vi "Execute.vi"(5 "SleepTerminalArray":refnum<vi>, 6 "ExeRef":refnum<vi>, 7 "ActiveTerminalArray":refnum<vi>, 8 "error in (no error)":errorcluster, 9 "Json_In":string, 10 "VariableRef":T2, 11 "Info":T1) -> (0 "Error Out":errorcluster, 1 "NumResultArray":dbl[](array[numeric]), 2 "StrResultArray":string[](array[string]), 3 "StrResult":string, 4 "NumResult":dbl)   [LabVIEW 2018, in "String.lvlib"]
uses:
  String.lvlib
  <userlib>/_OpenG.lib/dictionary/dictionary.llb/Dictionary Object RefNum__ogtk.ctl
  <userlib>/_OpenG.lib/dictionary/dictionary.llb/Dictionary Object RefNum - Enum__ogtk.ctl
  <vilib>/Utility/error.llb/whitespace.ctl
  <userlib>/_OpenG.lib/md5/md5.llb/MD5 Message Digest (Hexadecimal String)__ogtk.vi
  <vilib>/regexp/Match Regular Expression.xnode
  <vilib>/addons/_JKI.lib/Serialization/JSON/JKI JSON Serialization.lvlib
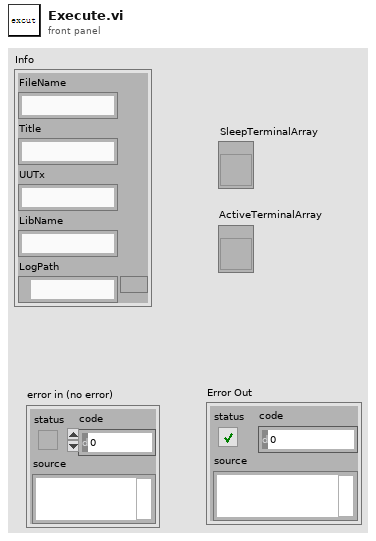
[diagram p1: front panel]
types:
  T1 = cluster{"FileName":string, "Title":string, "UUTx":string, "LibName":string, "LogPath":path}
  T2 = typedef "Dictionary Object RefNum__ogtk.ctl" = refnum<k1>
  T3 = cluster{"StringLength":cluster{"json":cluster{"Method":string, "StringVar":string}}, "InitialString":cluster{"json":cluster{"Method":string, "Strings":string}}, "StringSubset":cluster{"json":cluster{"Method":string, "StringVar":string, "offset":i32, "length":i32}}, "TrimWhitespace":cluster{"json":cluster{"Method":string, "StringVar":string, "Location":string}}, "ReplaceSubstring":cluster{"json":cluster{"Method":string, "StringVar":string, "Substring":string, "Offset":i32, "Length":i32}}, "SearchandReplaceString":cluster{"json":cluster{"Method":string, "StringVar":string, "SearchString":string, "Offset":i32, "ReplaceString":string, "ReplaceAll":bool, "IgnoreCase":bool}}, "MatchPattern":cluster{"json":cluster{"Method":string, "StringVar":string, "RegularExpression ":string, "Offset":i32}}, "MatchRegularExpression":cluster{"json":cluster{"Method":string, "StringVar":string, "RegularExpression ":string, "Offset":i32, "IgnoreCase":bool, "Multiline":bool}}, "FormatDate/TimeString":cluster{"json":cluster{"Method":string, "TimeFormatString ":string, "UTCFormat":bool}}, "ToLowerCase":cluster{"json":cluster{"Method":string, "StringVar":string}}, "ToUpperCase":cluster{"json":cluster{"Method":string, "StringVar":string}}, "StringMD5":cluster{"json":cluster{"Method":string, "StringVar":string}}, "NumStringToHexString":cluster{"json":cluster{"Method":string, "StringVar":string}}, "HexStringToNumString":cluster{"json":cluster{"Method":string, "StringVar":string}}, "StartWith":cluster{"json":cluster{"Method":string, "StringVar":string, "SubString":string, "IgnoreCasse":bool}}, "EndWith":cluster{"json":cluster{"Method":string, "StringVar":string, "SubString":string, "IgnoreCasse":bool}}, "AfterSubstring":cluster{"json":cluster{"Method":string, "StringVar":string, "SubString":string}}, "BeforeSubstring":cluster{"json":cluster{"Method":string, "StringVar":string, "SubString":string}}, "MiddleSubstring":cluster{"json":cluster{"Method":string, "StringVar":string, "BeforeSubString":string, "AfterSubString":string}}, "AsciiToHexString":cluster{"json":cluster{"Method":string, "StringVar":string}}, "HexStringToAscii":cluster{"json":cluster{"Method":string, "StringVar":string}}, "StringTo1DArray":cluster{"json":cluster{"Method":string, "StringVar":string, "Delimiter":string}}, "StringToCharacterArray":cluster{"json":cluster{"Method":string, "StringVar":string}}, "RemoveAllWhitespace":cluster{"json":cluster{"Method":string, "StringVar":string}}}
  T4 = cluster{"json":cluster{"Method":string, "StringVar":string}}
  T5 = cluster{"json":cluster{"Method":string, "Strings":string}}
  T6 = cluster{"json":cluster{"Method":string, "StringVar":string, "offset":i32, "length":i32}}
  T7 = cluster{"json":cluster{"Method":string, "StringVar":string, "Location":string}}
  T8 = typedef "whitespace.ctl" = u16
  T9 = cluster{"json":cluster{"Method":string, "StringVar":string, "Substring":string, "Offset":i32, "Length":i32}}
  T10 = cluster{"json":cluster{"Method":string, "StringVar":string, "SearchString":string, "Offset":i32, "ReplaceString":string, "ReplaceAll":bool, "IgnoreCase":bool}}
  T11 = cluster{"json":cluster{"Method":string, "StringVar":string, "RegularExpression ":string, "Offset":i32}}
  T12 = cluster{"json":cluster{"Method":string, "StringVar":string, "RegularExpression ":string, "Offset":i32, "IgnoreCase":bool, "Multiline":bool}}
  T13 = cluster{"json":cluster{"Method":string, "TimeFormatString ":string, "UTCFormat":bool}}
  T14 = cluster{"json":cluster{"Method":string, "StringVar":string, "SubString":string, "IgnoreCasse":bool}}
  T15 = cluster{"json":cluster{"Method":string, "StringVar":string, "SubString":string}}
  T16 = cluster{"json":cluster{"Method":string, "StringVar":string, "BeforeSubString":string, "AfterSubString":string}}
  T17 = cluster{"json":cluster{"Method":string, "StringVar":string, "Delimiter":string}}
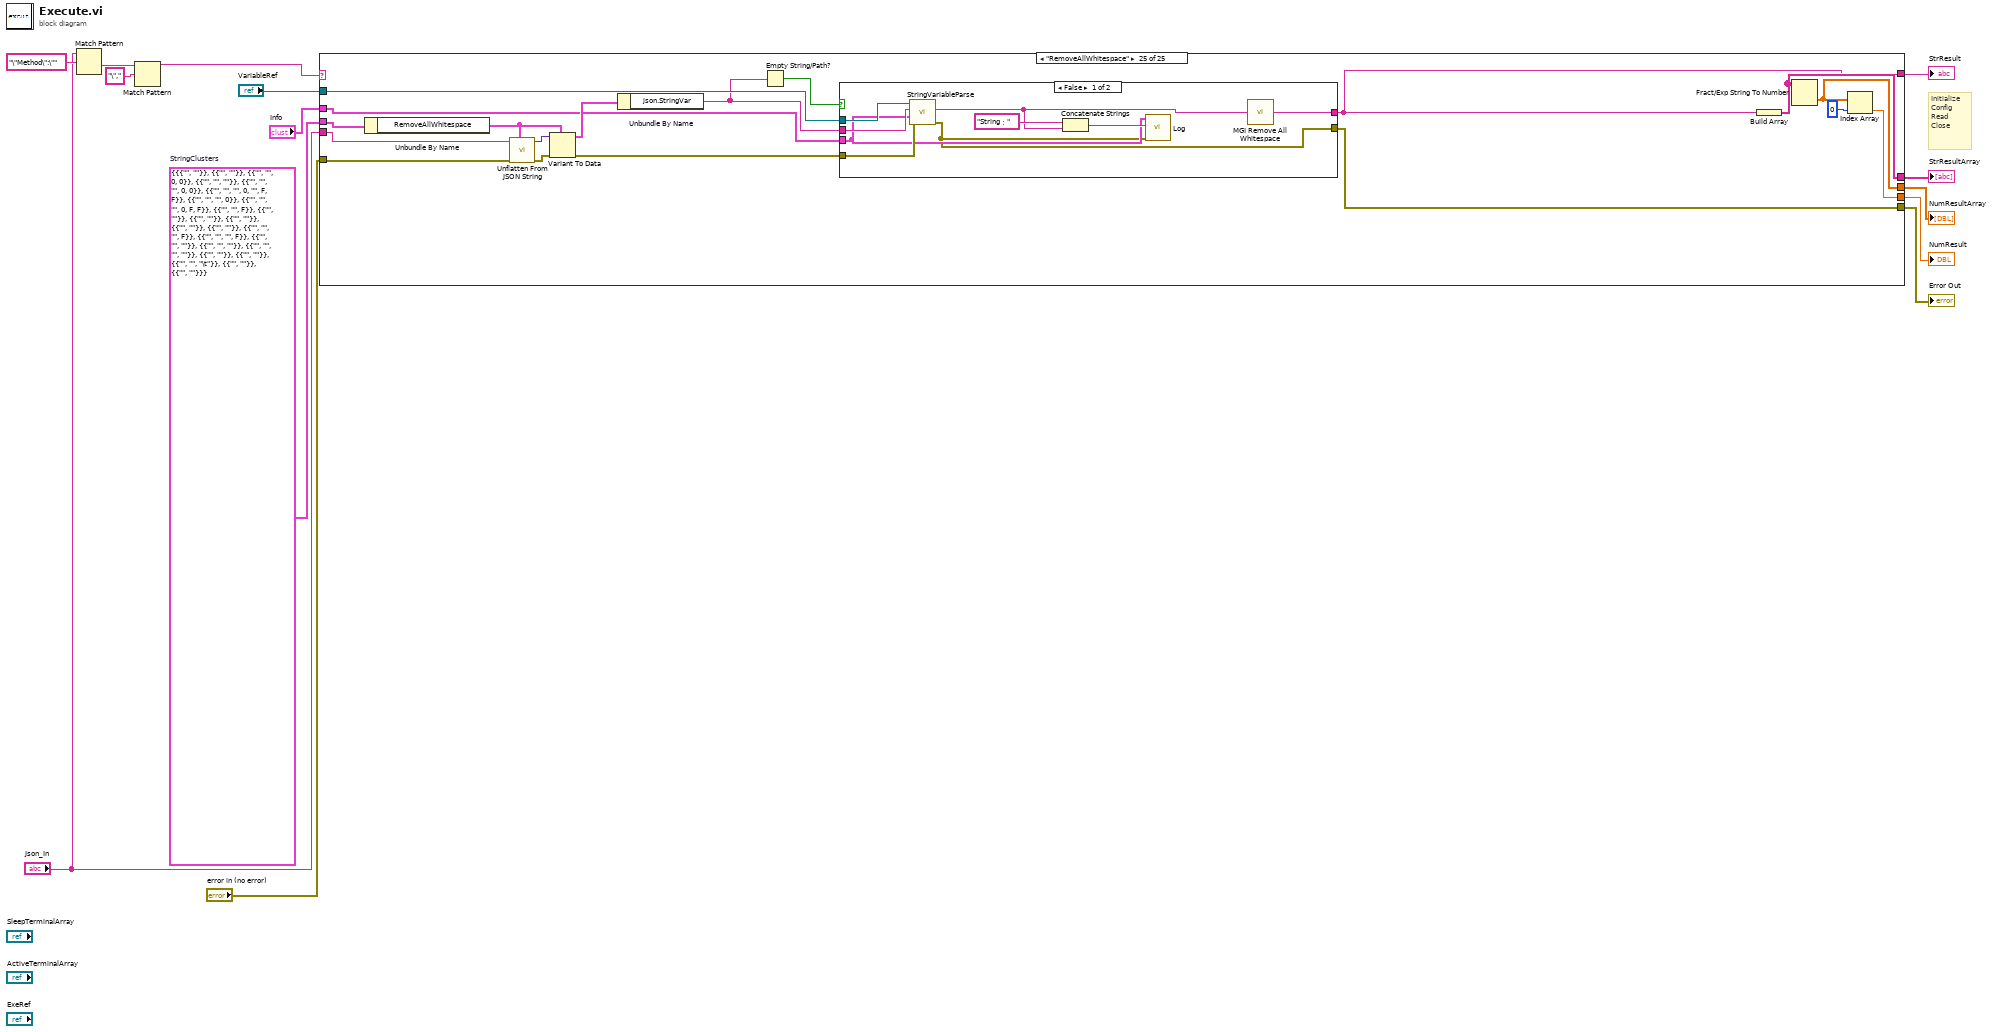
[diagram p0: block diagram]
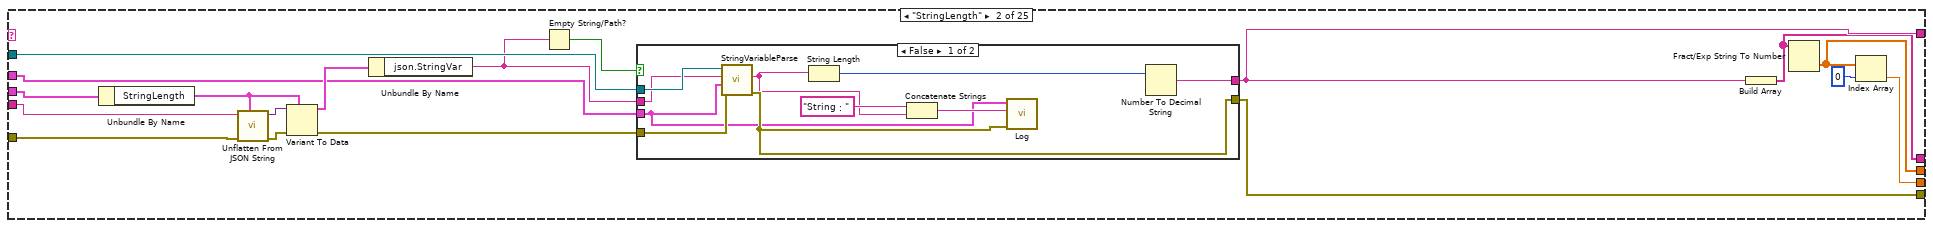
[diagram p3: hidden frame]
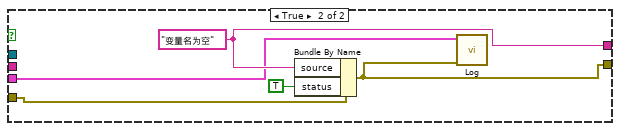
[diagram p4: hidden frame]
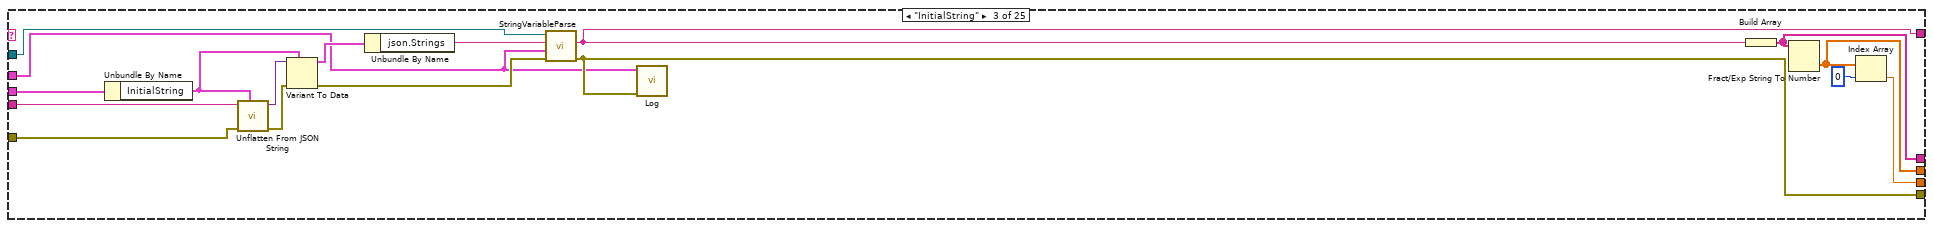
[diagram p5: hidden frame]
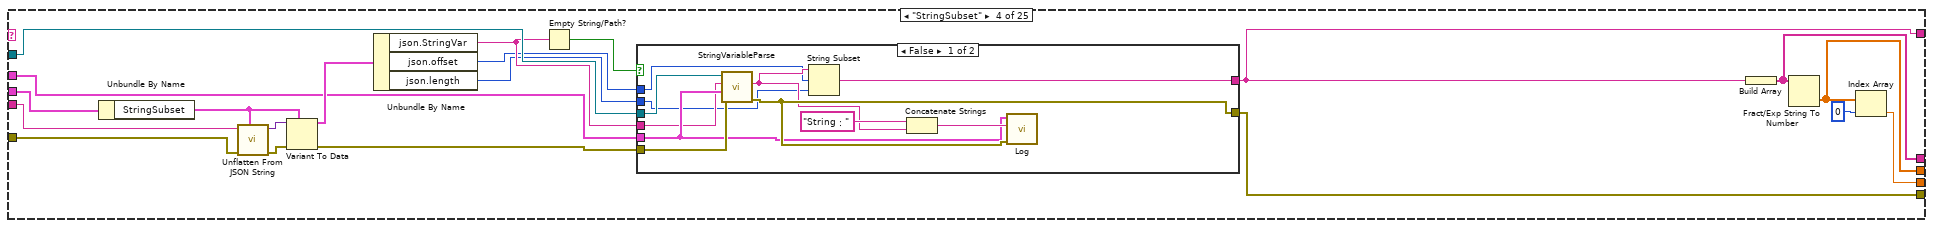
[diagram p6: hidden frame]
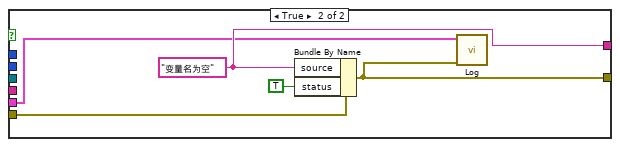
[diagram p7: hidden frame]
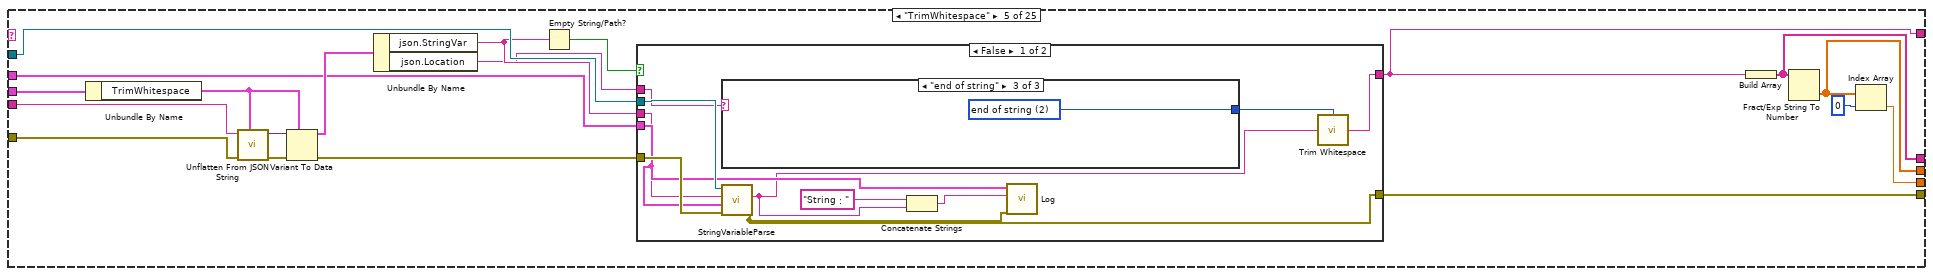
[diagram p8: hidden frame]
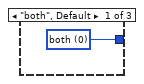
[diagram p9: hidden frame]
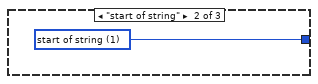
[diagram p10: hidden frame]
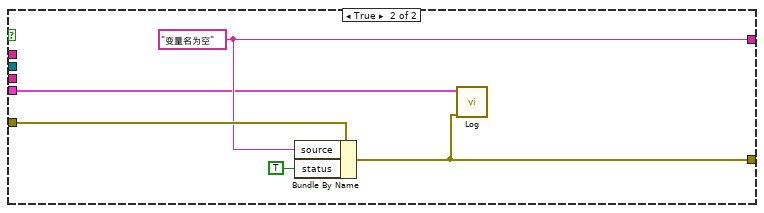
[diagram p11: hidden frame]
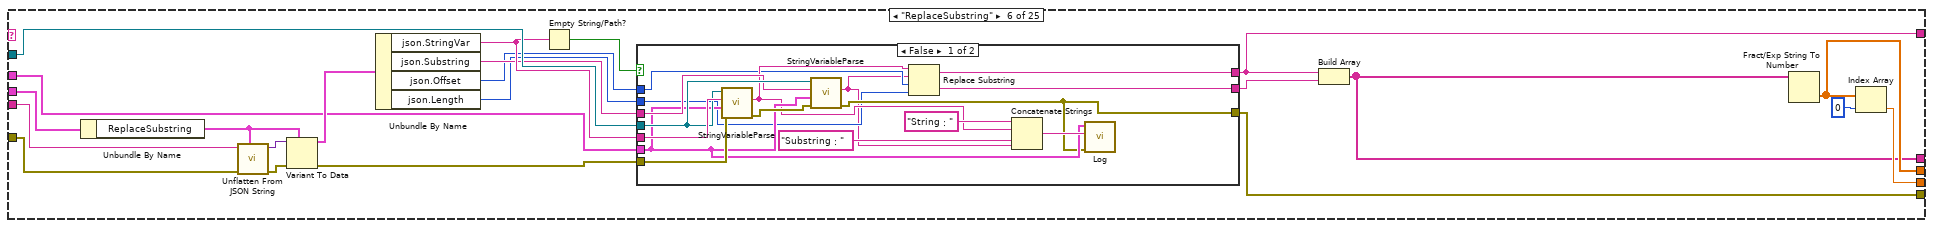
[diagram p12: hidden frame]
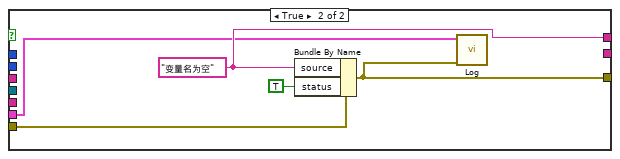
[diagram p13: hidden frame]
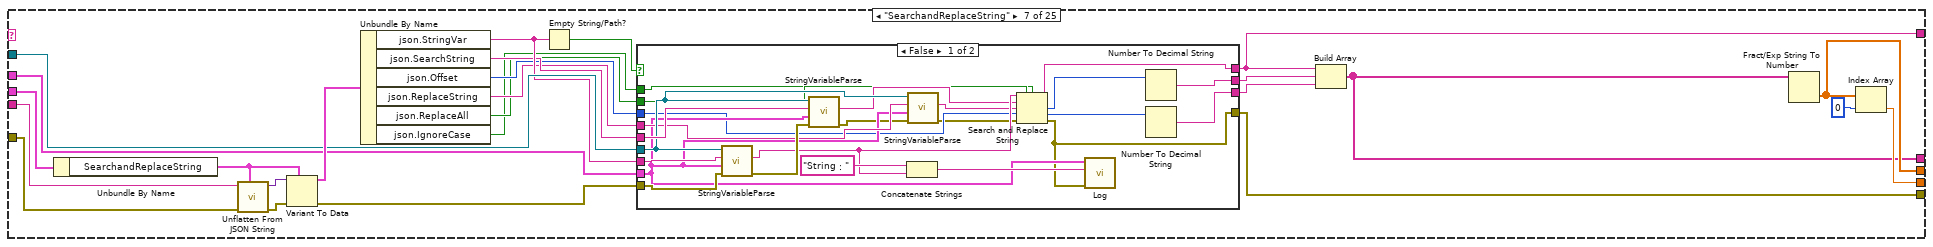
[diagram p14: hidden frame]
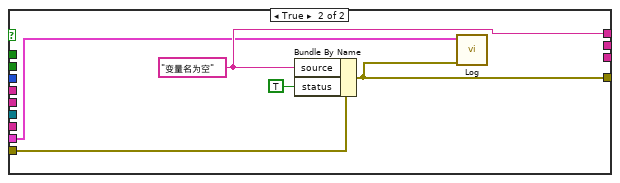
[diagram p15: hidden frame]
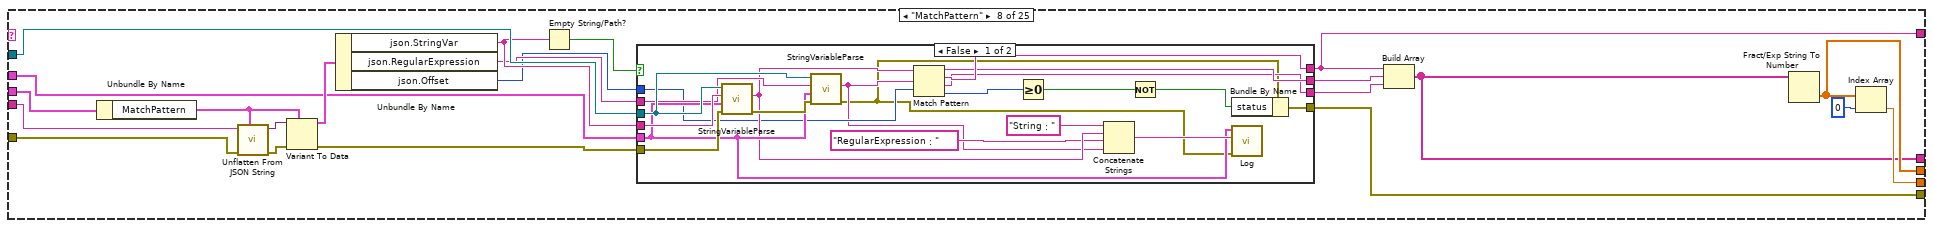
[diagram p16: hidden frame]
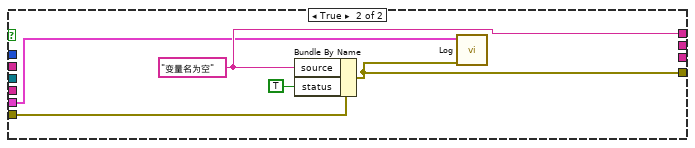
[diagram p17: hidden frame]
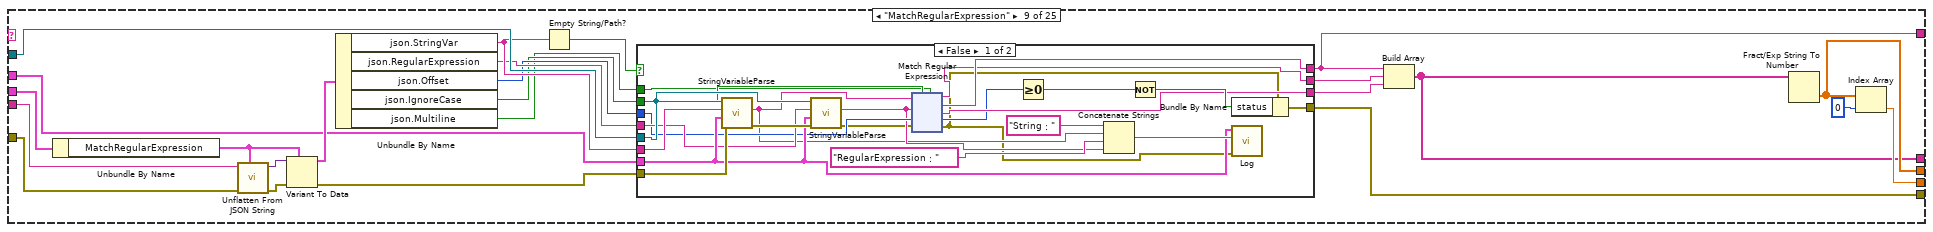
[diagram p18: hidden frame]
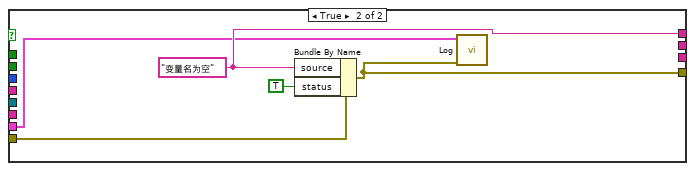
[diagram p19: hidden frame]
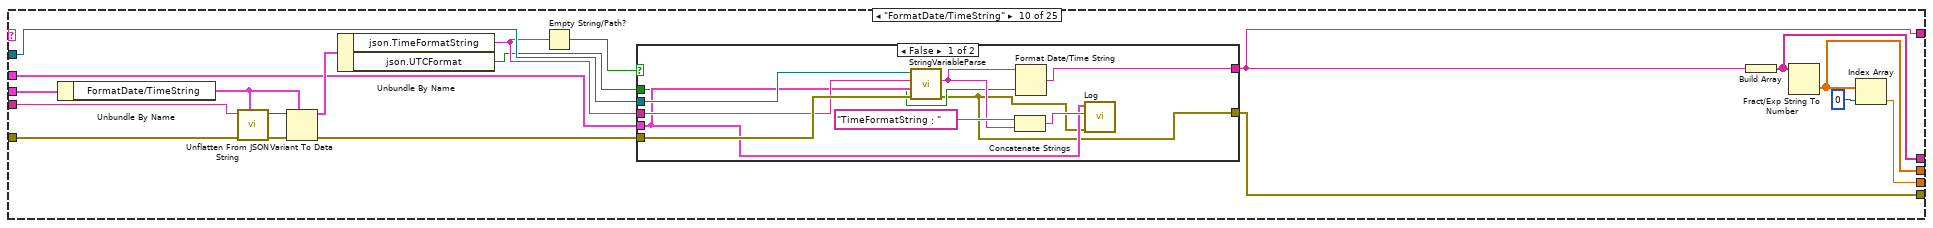
[diagram p20: hidden frame]
diagram:
  w1 = T3 {"StringLength"={"json"={"Method"="", "StringVar"=""}}, "InitialString"={"json"={"Method"="", "Strings"=""}}, "StringSubset"={"json"={"Method"="", "StringVar"="", "offset"=0, "length"=0}}, "TrimWhitespace"={"json"={"Method"="", "StringVar"="", "Location"=""}}, "ReplaceSubstring"={"json"={"Method"="", "StringVar"="", "Substring"="", "Offset"=0, "Length"=0}}, "SearchandReplaceString"={"json"={"Method"="", "StringVar"="", "SearchString"="", "Offset"=0, "ReplaceString"="", "ReplaceAll"=FALSE, "IgnoreCase"=FALSE}}, "MatchPattern"={"json"={"Method"="", "StringVar"="", "RegularExpression "="", "Offset"=0}}, "MatchRegularExpression"={"json"={"Method"="", "StringVar"="", "RegularExpression "="", "Offset"=0, "IgnoreCase"=FALSE, "Multiline"=FALSE}}, "FormatDate/TimeString"={"json"={"Method"="", "TimeFormatString "="", "UTCFormat"=FALSE}}, "ToLowerCase"={"json"={"Method"="", "StringVar"=""}}, "ToUpperCase"={"json"={"Method"="", "StringVar"=""}}, "StringMD5"={"json"={"Method"="", "StringVar"=""}}, "NumStringToHexString"={"json"={"Method"="", "StringVar"=""}}, "HexStringToNumString"={"json"={"Method"="", "StringVar"=""}}, "StartWith"={"json"={"Method"="", "StringVar"="", "SubString"="", "IgnoreCasse"=FALSE}}, "EndWith"={"json"={"Method"="", "StringVar"="", "SubString"="", "IgnoreCasse"=FALSE}}, "AfterSubstring"={"json"={"Method"="", "StringVar"="", "SubString"=""}}, "BeforeSubstring"={"json"={"Method"="", "StringVar"="", "SubString"=""}}, "MiddleSubstring"={"json"={"Method"="", "StringVar"="", "BeforeSubString"="", "AfterSubString"=""}}, "AsciiToHexString"={"json"={"Method"="", "StringVar"=""}}, "HexStringToAscii"={"json"={"Method"="", "StringVar"=""}}, "StringTo1DArray"={"json"={"Method"="", "StringVar"="", "Delimiter"="\t"}}, "StringToCharacterArray"={"json"={"Method"="", "StringVar"=""}}, "RemoveAllWhitespace"={"json"={"Method"="", "StringVar"=""}}}  # StringClusters
  # "Initialize\nConfig\nRead\nClose"
  n1 = Match Pattern(string="Json_In", regular expression="\"Method\":\"") -> (after substring=w4:string)  [unwired: 1 in, 3 out]
  n2 = Match Pattern(string=w4, regular expression="\",") -> (before substring=w2:string)  [unwired: 1 in, 3 out]
  n3 = case shown="\"RemoveAllWhitespace\"" w2 {
    tunnel: "Json_In" -> [_ w30 w62 w82 w117 w158 w204 w254 w303 w464 w497 w529 w561 w593 w626 w661 w821 w980 w1016 w1053 w1103 w1150 w1194 w1231 w1264]
    tunnel: [w15 w25 w58 w66 w102 w144 w190 w240 w289 w450 w483 w515 w547 w579 w612 w647 w807 w966 w1004 w1041 w1091 w1138 w1182 w1219 w1252] -> w14
    tunnel: "error in (no error)" -> [w15 w29 w61 w81 w116 w157 w203 w253 w302 w463 w496 w528 w560 w592 w625 w660 w820 w979 w1015 w1052 w1102 w1149 w1193 w1230 w1263]
    tunnel: [_ w17 w49 w67 w103 w145 w191 w241 w290 w451 w484 w516 w548 w580 w613 w648 w808 w967 w1002 w1037 w1089 w1136 w1180 w1218 w1250] -> w12
    tunnel: "VariableRef" -> [_ w27 w59 w73 w108 w149 w195 w245 w294 w455 w488 w520 w552 w584 w617 w652 w812 w971 w1008 w1045 w1095 w1142 w1186 w1223 w1256]
    tunnel: [_ w16 w50 w75 w110 w151 w197 w247 w296 w457 w490 w522 w554 w586 w619 w654 w814 w973 w1001 w1038 w1090 w1137 w1179 w1217 w1251] -> w11
    tunnel: [_ w20 w53 w78 w113 w154 w200 w250 w299 w460 w493 w525 w557 w589 w622 w657 w817 w976 w1012 w1049 w1099 w1146 w1190 w1227 w1260] -> w10
    tunnel: [_ w22 w55 w80 w115 w156 w202 w252 w301 w462 w495 w527 w559 w591 w624 w659 w819 w978 w1014 w1051 w1101 w1148 w1192 w1229 w1262] -> w9
    tunnel: "Info" -> [_ w23 w56 w70 w105 w146 w192 w242 w291 w452 w485 w517 w549 w581 w614 w649 w809 w968 w1005 w1042 w1092 w1139 w1183 w1220 w1253]
    tunnel: w1 -> [_ w19 w52 w77 w112 w153 w199 w249 w298 w459 w492 w524 w556 w588 w621 w656 w816 w975 w1011 w1048 w1098 w1145 w1189 w1226 w1259]
    frame Default {
    }
    frame "StringLength" {
      n4 = Unbundle By Name(w19) -> ("StringLength"=w18:T4)
      n5 = call <vilib>:"Unflatten From JSON String.vi"("Type and Defaults"=w18, "error in (no error)"=w29, "JSON String"=w30) -> ("error out"=w32:errorcluster, "Variant"=w33:variant)  [unwired: 7 in]
      n6 = Variant To Data(error in=w32, type=w18, Variant=w33) -> (data=w31:T4, error out=w28:errorcluster)
      n7 = Unbundle By Name(w31) -> ("json.StringVar"=w24:string)
      n8 = Empty String/Path?(string/path=w24) -> (empty?=w26:bool)
      n9 = case shown="False" w26 {
        tunnel: w28 -> [w43 w48]
        tunnel: w27 -> [w42 _]
        tunnel: [w41 w44] -> w25
        tunnel: w24 -> [w38 _]
        tunnel: [w34 w46] -> w17
        tunnel: w23 -> [w39 w45]
        frame False {
          n10 = call "StringVariableParse.vi"("error in"=w43, "Info"=w39, "in"=w38, "dictionary"=w42) -> ("error out"=w41:errorcluster, "out"=w36:string)  [unwired: 5 in, 1 out]
          n11 = String Length(string=w36) -> (length=w35:i32)
          n12 = Concatenate Strings("String：" ("string"), w36) -> (w40:string)
          n13 = call "Log.vi"("error in"=w41, "LogIn"=w40, "Info"=w39) -> ()  [unwired: 9 in]
          n14 = Number To Decimal String(number=w35) -> (decimal integer string=w34:string)  [unwired: 1 in]
        }
        frame True {
          w46 = "变量名为空" ("source")
          n15 = Bundle By Name(cluster=w48, "source"=w46, "status"=TRUE) -> (w44:errorcluster)
          n16 = call "Log.vi"("error in"=w44, "Info"=w45) -> ()  [unwired: 10 in]
        }
      }
      n17 = Build Array(w17) -> (w16:string[])
      n18 = Fract/Exp String To Number(string=w16) -> (number=w22:dbl[])  [unwired: 3 in, 1 out]
      n19 = Index Array(array=w22, index=0) -> (element=w20:dbl)
    }
    frame "InitialString" {
      n20 = Unbundle By Name(w52) -> ("InitialString"=w51:T5)
      n21 = call <vilib>:"Unflatten From JSON String.vi"("Type and Defaults"=w51, "error in (no error)"=w61, "JSON String"=w62) -> ("error out"=w64:errorcluster, "Variant"=w65:variant)  [unwired: 7 in]
      n22 = Variant To Data(error in=w64, type=w51, Variant=w65) -> (data=w63:T5, error out=w60:errorcluster)
      n23 = Unbundle By Name(w63) -> ("json.Strings"=w57:string)
      n24 = call "StringVariableParse.vi"("error in"=w60, "Info"=w56, "in"=w57, "dictionary"=w59) -> ("error out"=w58:errorcluster, "out"=w49:string)  [unwired: 5 in, 1 out]
      n25 = call "Log.vi"("error in"=w58, "Info"=w56) -> ()  [unwired: 10 in]
      n26 = Build Array(w49) -> (w50:string[])
      n27 = Fract/Exp String To Number(string=w50) -> (number=w55:dbl[])  [unwired: 3 in, 1 out]
      n28 = Index Array(array=w55, index=0) -> (element=w53:dbl)
    }
    frame "StringSubset" {
      n29 = Unbundle By Name(w77) -> ("StringSubset"=w76:T6)
      n30 = call <vilib>:"Unflatten From JSON String.vi"("Type and Defaults"=w76, "error in (no error)"=w81, "JSON String"=w82) -> ("error out"=w84:errorcluster, "Variant"=w85:variant)  [unwired: 7 in]
      n31 = Variant To Data(error in=w84, type=w76, Variant=w85) -> (data=w83:T6, error out=w71:errorcluster)
      n32 = Unbundle By Name(w83) -> ("json.StringVar"=w72:string, "json.offset"=w69:i32, "json.length"=w68:i32)
      n33 = Empty String/Path?(string/path=w72) -> (empty?=w74:bool)
      n34 = case shown="False" w74 {
        tunnel: w71 -> [w96 w101]
        tunnel: w73 -> [w95 _]
        tunnel: [w94 w97] -> w66
        tunnel: w72 -> [w91 _]
        tunnel: [w86 w99] -> w67
        tunnel: w70 -> [w92 w98]
        tunnel: w69 -> [w88 _]
        tunnel: w68 -> [w87 _]
        frame False {
          n35 = call "StringVariableParse.vi"("error in"=w96, "Info"=w92, "in"=w91, "dictionary"=w95) -> ("error out"=w94:errorcluster, "out"=w89:string)  [unwired: 5 in, 1 out]
          n36 = String Subset(string=w89, offset (0)=w88, length (rest)=w87) -> (substring=w86:string)
          n37 = Concatenate Strings("String：" ("string"), w89) -> (w93:string)
          n38 = call "Log.vi"("error in"=w94, "LogIn"=w93, "Info"=w92) -> ()  [unwired: 9 in]
        }
        frame True {
          w99 = "变量名为空" ("source")
          n39 = Bundle By Name(cluster=w101, "source"=w99, "status"=TRUE) -> (w97:errorcluster)
          n40 = call "Log.vi"("error in"=w97, "Info"=w98) -> ()  [unwired: 10 in]
        }
      }
      n41 = Build Array(w67) -> (w75:string[])
      n42 = Fract/Exp String To Number(string=w75) -> (number=w80:dbl[])  [unwired: 3 in, 1 out]
      n43 = Index Array(array=w80, index=0) -> (element=w78:dbl)
    }
    frame "TrimWhitespace" {
      n44 = Unbundle By Name(w112) -> ("TrimWhitespace"=w111:T7)
      n45 = call <vilib>:"Unflatten From JSON String.vi"("Type and Defaults"=w111, "error in (no error)"=w116, "JSON String"=w117) -> ("error out"=w119:errorcluster, "Variant"=w120:variant)  [unwired: 7 in]
      n46 = Variant To Data(error in=w119, type=w111, Variant=w120) -> (data=w118:T7, error out=w106:errorcluster)
      n47 = Unbundle By Name(w118) -> ("json.StringVar"=w107:string, "json.Location"=w104:string)
      n48 = Empty String/Path?(string/path=w107) -> (empty?=w109:bool)
      n49 = case shown="False" w109 {
        tunnel: w106 -> [w131 w139]
        tunnel: w108 -> [w130 _]
        tunnel: [w129 w135] -> w102
        tunnel: w107 -> [w126 _]
        tunnel: [w124 w137] -> w103
        tunnel: w105 -> [w127 w136]
        tunnel: w104 -> [w121 _]
        frame False {
          n50 = case shown="\"end of string\"" w121 {
            tunnel: [w132 w133 w134] -> w122
            frame "both", Default {
              w132 = T8 0 items=["both", "start of string", "end of string"] ("location (both)")
            }
            frame "start of string" {
              w133 = T8 1 items=["both", "start of string", "end of string"] ("location (both)")
            }
            frame "end of string" {
              w134 = T8 2 items=["both", "start of string", "end of string"] ("location (both)")
            }
          }
          n51 = call "StringVariableParse.vi"("error in"=w131, "Info"=w127, "in"=w126, "dictionary"=w130) -> ("error out"=w129:errorcluster, "out"=w123:string)  [unwired: 5 in, 1 out]
          n52 = Concatenate Strings("String：" ("string"), w123) -> (w128:string)
          n53 = call "Log.vi"("error in"=w129, "LogIn"=w128, "Info"=w127) -> ()  [unwired: 9 in]
          n54 = call <vilib>:"Trim Whitespace.vi"("string"=w123, "location (both)"=w122) -> ("trimmed string"=w124:string)
        }
        frame True {
          w137 = "变量名为空" ("source")
          n55 = Bundle By Name(cluster=w139, "source"=w137, "status"=TRUE) -> (w135:errorcluster)
          n56 = call "Log.vi"("error in"=w135, "Info"=w136) -> ()  [unwired: 10 in]
        }
      }
      n57 = Build Array(w103) -> (w110:string[])
      n58 = Fract/Exp String To Number(string=w110) -> (number=w115:dbl[])  [unwired: 3 in, 1 out]
      n59 = Index Array(array=w115, index=0) -> (element=w113:dbl)
    }
    frame "ReplaceSubstring" {
      n60 = Unbundle By Name(w153) -> ("ReplaceSubstring"=w152:T9)
      n61 = call <vilib>:"Unflatten From JSON String.vi"("Type and Defaults"=w152, "error in (no error)"=w157, "JSON String"=w158) -> ("error out"=w160:errorcluster, "Variant"=w161:variant)  [unwired: 7 in]
      n62 = Variant To Data(error in=w160, type=w152, Variant=w161) -> (data=w159:T9, error out=w147:errorcluster)
      n63 = Unbundle By Name(w159) -> ("json.StringVar"=w148:string, "json.Substring"=w143:string, "json.Offset"=w142:i32, "json.Length"=w141:i32)
      n64 = Empty String/Path?(string/path=w148) -> (empty?=w150:bool)
      n65 = case shown="False" w150 {
        tunnel: w147 -> [w177 w182]
        tunnel: w149 -> [w172 _]
        tunnel: [w169 w178] -> w144
        tunnel: w148 -> [w175 _]
        tunnel: [w165 w180] -> w145
        tunnel: w146 -> [w170 w179]
        tunnel: w143 -> [w171 _]
        tunnel: w142 -> [w167 _]
        tunnel: w141 -> [w166 _]
        tunnel: [w162 _] -> w140
        frame False {
          n66 = call "StringVariableParse.vi"("error in"=w177, "Info"=w170, "in"=w175, "dictionary"=w172) -> ("error out"=w173:errorcluster, "out"=w168:string)  [unwired: 5 in, 1 out]
          n67 = call "StringVariableParse.vi"("error in"=w173, "Info"=w170, "in"=w171, "dictionary"=w172) -> ("error out"=w169:errorcluster, "out"=w163:string)  [unwired: 5 in, 1 out]
          n68 = Replace Substring(2:w166, 3:w167, 4:w163, 5:w168) -> (0:w162:string, 1:w165:string)
          n69 = Concatenate Strings("String：" ("string"), w168, "Substring：" ("string"), w163) -> (w176:string)
          n70 = call "Log.vi"("error in"=w169, "LogIn"=w176, "Info"=w170) -> ()  [unwired: 9 in]
        }
        frame True {
          w180 = "变量名为空" ("source")
          n71 = Bundle By Name(cluster=w182, "source"=w180, "status"=TRUE) -> (w178:errorcluster)
          n72 = call "Log.vi"("error in"=w178, "Info"=w179) -> ()  [unwired: 10 in]
        }
      }
      n73 = Build Array(w145, w140) -> (w151:string[])
      n74 = Fract/Exp String To Number(string=w151) -> (number=w156:dbl[])  [unwired: 3 in, 1 out]
      n75 = Index Array(array=w156, index=0) -> (element=w154:dbl)
    }
    frame "SearchandReplaceString" {
      n76 = Unbundle By Name(w199) -> ("SearchandReplaceString"=w198:T10)
      n77 = call <vilib>:"Unflatten From JSON String.vi"("Type and Defaults"=w198, "error in (no error)"=w203, "JSON String"=w204) -> ("error out"=w206:errorcluster, "Variant"=w207:variant)  [unwired: 7 in]
      n78 = Variant To Data(error in=w206, type=w198, Variant=w207) -> (data=w205:T10, error out=w193:errorcluster)
      n79 = Unbundle By Name(w205) -> ("json.StringVar"=w194:string, "json.SearchString"=w189:string, "json.Offset"=w188:i32, "json.ReplaceString"=w187:string, "json.ReplaceAll"=w186:bool, "json.IgnoreCase"=w185:bool)
      n80 = Empty String/Path?(string/path=w194) -> (empty?=w196:bool)
      n81 = case shown="False" w196 {
        tunnel: w193 -> [w230 w235]
        tunnel: w195 -> [w224 _]
        tunnel: [w212 w231] -> w190
        tunnel: w194 -> [w228 _]
        tunnel: [w214 w233] -> w191
        tunnel: w192 -> [w222 w232]
        tunnel: w189 -> [w225 _]
        tunnel: w188 -> [w217 _]
        tunnel: w187 -> [w223 _]
        tunnel: w186 -> [w216 _]
        tunnel: w185 -> [w215 _]
        tunnel: [w209 _] -> w184
        tunnel: [w208 _] -> w183
        frame False {
          n82 = call "StringVariableParse.vi"("error in"=w230, "Info"=w222, "in"=w228, "dictionary"=w224) -> ("error out"=w226:errorcluster, "out"=w220:string)  [unwired: 5 in, 1 out]
          n83 = call "StringVariableParse.vi"("error in"=w226, "Info"=w222, "in"=w225, "dictionary"=w224) -> ("error out"=w221:errorcluster, "out"=w219:string)  [unwired: 5 in, 1 out]
          n84 = Concatenate Strings("String：" ("string"), w220) -> (w229:string)
          n85 = call "StringVariableParse.vi"("error in"=w221, "Info"=w222, "in"=w223, "dictionary"=w224) -> ("error out"=w213:errorcluster, "out"=w218:string)  [unwired: 5 in, 1 out]
          n86 = Search and Replace String(replace all?=w216, case sensitive?=w215, input string=w220, search string=w219, replace string=w218, offset=w217, error in=w213) -> (result string=w214:string, number of replacements=w211:i32, offset past replacement=w210:i32, error out=w212:errorcluster)  [unwired: 1 in]
          n87 = call "Log.vi"("error in"=w212, "LogIn"=w229, "Info"=w222) -> ()  [unwired: 9 in]
          n88 = Number To Decimal String(number=w211) -> (decimal integer string=w209:string)  [unwired: 1 in]
          n89 = Number To Decimal String(number=w210) -> (decimal integer string=w208:string)  [unwired: 1 in]
        }
        frame True {
          w233 = "变量名为空" ("source")
          n90 = Bundle By Name(cluster=w235, "source"=w233, "status"=TRUE) -> (w231:errorcluster)
          n91 = call "Log.vi"("error in"=w231, "Info"=w232) -> ()  [unwired: 10 in]
        }
      }
      n92 = Build Array(w191, w184, w183) -> (w197:string[])
      n93 = Fract/Exp String To Number(string=w197) -> (number=w202:dbl[])  [unwired: 3 in, 1 out]
      n94 = Index Array(array=w202, index=0) -> (element=w200:dbl)
    }
    frame "MatchPattern" {
      n95 = Unbundle By Name(w249) -> ("MatchPattern"=w248:T11)
      n96 = call <vilib>:"Unflatten From JSON String.vi"("Type and Defaults"=w248, "error in (no error)"=w253, "JSON String"=w254) -> ("error out"=w256:errorcluster, "Variant"=w257:variant)  [unwired: 7 in]
      n97 = Variant To Data(error in=w256, type=w248, Variant=w257) -> (data=w255:T11, error out=w243:errorcluster)
      n98 = Unbundle By Name(w255) -> ("json.StringVar"=w244:string, "json.RegularExpression"=w237:string, "json.Offset"=w236:i32)
      n99 = Empty String/Path?(string/path=w244) -> (empty?=w246:bool)
      n100 = case shown="False" w246 {
        tunnel: w243 -> [w277 w282]
        tunnel: w245 -> [w272 _]
        tunnel: [w266 w278] -> w240
        tunnel: w244 -> [w275 _]
        tunnel: [w263 w280] -> w241
        tunnel: w242 -> [w271 w279]
        tunnel: [w262 _] -> w239
        tunnel: [w261 _] -> w238
        tunnel: w237 -> [w270 _]
        tunnel: w236 -> [w268 _]
        frame False {
          n101 = call "StringVariableParse.vi"("error in"=w277, "Info"=w271, "in"=w275, "dictionary"=w272) -> ("error out"=w273:errorcluster, "out"=w269:string)  [unwired: 5 in, 1 out]
          n102 = call "StringVariableParse.vi"("error in"=w273, "Info"=w271, "in"=w270, "dictionary"=w272) -> ("error out"=w258:errorcluster, "out"=w259:string)  [unwired: 5 in, 1 out]
          n103 = Match Pattern(string=w269, regular expression=w259, offset (0)=w268) -> (before substring=w262:string, match substring=w263:string, after substring=w261:string, offset past match=w267:i32)
          n104 = Greater Or Equal To 0?(x=w267) -> (x >= 0?=w265:bool)
          n105 = Concatenate Strings("String：" ("string"), w269, "RegularExpression：" ("string"), w259) -> (w276:string)
          n106 = Not(x=w265) -> (.not. x?=w264:bool)
          n107 = Bundle By Name(cluster=w258, "status"=w264) -> (w266:errorcluster)
          n108 = call "Log.vi"("error in"=w258, "LogIn"=w276, "Info"=w271) -> ()  [unwired: 9 in]
        }
        frame True {
          w280 = "变量名为空" ("source")
          n109 = Bundle By Name(cluster=w282, "source"=w280, "status"=TRUE) -> (w278:errorcluster)
          n110 = call "Log.vi"("error in"=w278, "Info"=w279) -> ()  [unwired: 10 in]
        }
      }
      n111 = Build Array(w241, w239, w238) -> (w247:string[])
      n112 = Fract/Exp String To Number(string=w247) -> (number=w252:dbl[])  [unwired: 3 in, 1 out]
      n113 = Index Array(array=w252, index=0) -> (element=w250:dbl)
    }
    frame "MatchRegularExpression" {
      n114 = Unbundle By Name(w298) -> ("MatchRegularExpression"=w297:T12)
      n115 = call <vilib>:"Unflatten From JSON String.vi"("Type and Defaults"=w297, "error in (no error)"=w302, "JSON String"=w303) -> ("error out"=w305:errorcluster, "Variant"=w306:variant)  [unwired: 7 in]
      n116 = Variant To Data(error in=w305, type=w297, Variant=w306) -> (data=w304:T12, error out=w292:errorcluster)
      n117 = Unbundle By Name(w304) -> ("json.StringVar"=w293:string, "json.RegularExpression"=w286:string, "json.Offset"=w285:i32, "json.IgnoreCase"=w284:bool, "json.Multiline"=w283:bool)
      n118 = Empty String/Path?(string/path=w293) -> (empty?=w295:bool)
      n119 = case shown="False" w295 {
        tunnel: w292 -> [w329 w448]
        tunnel: w294 -> [w324 _]
        tunnel: [w320 w444] -> w289
        tunnel: w293 -> [w327 _]
        tunnel: [w317 w446] -> w290
        tunnel: w291 -> [w323 w445]
        tunnel: [w316 _] -> w288
        tunnel: [w315 _] -> w287
        tunnel: w286 -> [w322 _]
        tunnel: w285 -> [w321 _]
        tunnel: w284 -> [w310 _]
        tunnel: w283 -> [w309 _]
        frame False {
          n120 = call "StringVariableParse.vi"("error in"=w329, "Info"=w323, "in"=w327, "dictionary"=w324) -> ("error out"=w325:errorcluster, "out"=w312:string)  [unwired: 5 in, 1 out]
          n121 = call "StringVariableParse.vi"("error in"=w325, "Info"=w323, "in"=w322, "dictionary"=w324) -> ("error out"=w311:errorcluster, "out"=w313:string)  [unwired: 5 in, 1 out]
          n122 = xnode "Match Regular Expression"("input string"=w312, "regular expression"=w313, "offset (0)"=w321, "error in"=w311, "ignore case? (F)"=w310, "multiline? (F)"=w309) -> ("before match"=w316:string, "whole match"=w317:string, "after match"=w315:string, "offset past match"=w308:i32, "error out"=w307:errorcluster)
          n123 = Greater Or Equal To 0?(x=w308) -> (x >= 0?=w319:bool)
          n124 = Concatenate Strings("String：" ("string"), w312, "RegularExpression：" ("string"), w313) -> (w328:string)
          n125 = Not(x=w319) -> (.not. x?=w318:bool)
          n126 = Bundle By Name(cluster=w307, "status"=w318) -> (w320:errorcluster)
          n127 = call "Log.vi"("error in"=w307, "LogIn"=w328, "Info"=w323) -> ()  [unwired: 9 in]
        }
        frame True {
          w446 = "变量名为空" ("source")
          n128 = Bundle By Name(cluster=w448, "source"=w446, "status"=TRUE) -> (w444:errorcluster)
          n129 = call "Log.vi"("error in"=w444, "Info"=w445) -> ()  [unwired: 10 in]
        }
      }
      n130 = Build Array(w290, w288, w287) -> (w296:string[])
      n131 = Fract/Exp String To Number(string=w296) -> (number=w301:dbl[])  [unwired: 3 in, 1 out]
      n132 = Index Array(array=w301, index=0) -> (element=w299:dbl)
    }
    frame "FormatDate/TimeString" {
      n133 = Unbundle By Name(w459) -> ("FormatDate/TimeString"=w458:T13)
      n134 = call <vilib>:"Unflatten From JSON String.vi"("Type and Defaults"=w458, "error in (no error)"=w463, "JSON String"=w464) -> ("error out"=w466:errorcluster, "Variant"=w467:variant)  [unwired: 7 in]
      n135 = Variant To Data(error in=w466, type=w458, Variant=w467) -> (data=w465:T13, error out=w453:errorcluster)
      n136 = Unbundle By Name(w465) -> ("json.TimeFormatString"=w454:string, "json.UTCFormat"=w449:bool)
      n137 = Empty String/Path?(string/path=w454) -> (empty?=w456:bool)
      n138 = case shown="False" w456 {
        tunnel: w453 -> [w477 w482]
        tunnel: w455 -> [w473 _]
        tunnel: [w468 w478] -> w450
        tunnel: w454 -> [w475 _]
        tunnel: [w469 w480] -> w451
        tunnel: w452 -> [w472 w479]
        tunnel: w449 -> [w470 _]
        frame False {
          n139 = call "StringVariableParse.vi"("error in"=w477, "Info"=w472, "in"=w475, "dictionary"=w473) -> ("error out"=w468:errorcluster, "out"=w471:string)  [unwired: 5 in, 1 out]
          n140 = Concatenate Strings("TimeFormatString：" ("string"), w471) -> (w476:string)
          n141 = Format Date/Time String(time format string (%c)=w471, UTC format=w470) -> (date/time string=w469:string)  [unwired: 1 in]
          n142 = call "Log.vi"("error in"=w468, "LogIn"=w476, "Info"=w472) -> ()  [unwired: 9 in]
        }
        frame True {
          w480 = "变量名为空" ("source")
          n143 = Bundle By Name(cluster=w482, "source"=w480, "status"=TRUE) -> (w478:errorcluster)
          n144 = call "Log.vi"("error in"=w478, "Info"=w479) -> ()  [unwired: 10 in]
        }
      }
      n145 = Build Array(w451) -> (w457:string[])
      n146 = Fract/Exp String To Number(string=w457) -> (number=w462:dbl[])  [unwired: 3 in, 1 out]
      n147 = Index Array(array=w462, index=0) -> (element=w460:dbl)
    }
    frame "ToLowerCase" {
      n148 = Unbundle By Name(w492) -> ("ToLowerCase"=w491:T4)
      n149 = call <vilib>:"Unflatten From JSON String.vi"("Type and Defaults"=w491, "error in (no error)"=w496, "JSON String"=w497) -> ("error out"=w499:errorcluster, "Variant"=w500:variant)  [unwired: 7 in]
      n150 = Variant To Data(error in=w499, type=w491, Variant=w500) -> (data=w498:T4, error out=w486:errorcluster)
      n151 = Unbundle By Name(w498) -> ("json.StringVar"=w487:string)
      n152 = Empty String/Path?(string/path=w487) -> (empty?=w489:bool)
      n153 = case shown="False" w489 {
        tunnel: w486 -> [w509 w514]
        tunnel: w488 -> [w505 _]
        tunnel: [w501 w510] -> w483
        tunnel: w487 -> [w507 _]
        tunnel: [w503 w512] -> w484
        tunnel: w485 -> [w504 w511]
        frame False {
          n154 = call "StringVariableParse.vi"("error in"=w509, "Info"=w504, "in"=w507, "dictionary"=w505) -> ("error out"=w501:errorcluster, "out"=w502:string)  [unwired: 5 in, 1 out]
          n155 = Concatenate Strings("String：" ("string"), w502) -> (w508:string)
          n156 = call "Log.vi"("error in"=w501, "LogIn"=w508, "Info"=w504) -> ()  [unwired: 9 in]
          n157 = To Lower Case(string=w502) -> (all lower case string=w503:string)
        }
        frame True {
          w512 = "变量名为空" ("source")
          n158 = Bundle By Name(cluster=w514, "source"=w512, "status"=TRUE) -> (w510:errorcluster)
          n159 = call "Log.vi"("error in"=w510, "Info"=w511) -> ()  [unwired: 10 in]
        }
      }
      n160 = Build Array(w484) -> (w490:string[])
      n161 = Fract/Exp String To Number(string=w490) -> (number=w495:dbl[])  [unwired: 3 in, 1 out]
      n162 = Index Array(array=w495, index=0) -> (element=w493:dbl)
    }
    frame "ToUpperCase" {
      n163 = Unbundle By Name(w524) -> ("ToUpperCase"=w523:T4)
      n164 = call <vilib>:"Unflatten From JSON String.vi"("Type and Defaults"=w523, "error in (no error)"=w528, "JSON String"=w529) -> ("error out"=w531:errorcluster, "Variant"=w532:variant)  [unwired: 7 in]
      n165 = Variant To Data(error in=w531, type=w523, Variant=w532) -> (data=w530:T4, error out=w518:errorcluster)
      n166 = Unbundle By Name(w530) -> ("json.StringVar"=w519:string)
      n167 = Empty String/Path?(string/path=w519) -> (empty?=w521:bool)
      n168 = case shown="False" w521 {
        tunnel: w518 -> [w541 w546]
        tunnel: w520 -> [w537 _]
        tunnel: [w533 w542] -> w515
        tunnel: w519 -> [w539 _]
        tunnel: [w535 w544] -> w516
        tunnel: w517 -> [w536 w543]
        frame False {
          n169 = call "StringVariableParse.vi"("error in"=w541, "Info"=w536, "in"=w539, "dictionary"=w537) -> ("error out"=w533:errorcluster, "out"=w534:string)  [unwired: 5 in, 1 out]
          n170 = Concatenate Strings("String：" ("string"), w534) -> (w540:string)
          n171 = call "Log.vi"("error in"=w533, "LogIn"=w540, "Info"=w536) -> ()  [unwired: 9 in]
          n172 = To Upper Case(1:w534) -> (0:w535:string)
        }
        frame True {
          w544 = "变量名为空" ("source")
          n173 = Bundle By Name(cluster=w546, "source"=w544, "status"=TRUE) -> (w542:errorcluster)
          n174 = call "Log.vi"("error in"=w542, "Info"=w543) -> ()  [unwired: 10 in]
        }
      }
      n175 = Build Array(w516) -> (w522:string[])
      n176 = Fract/Exp String To Number(string=w522) -> (number=w527:dbl[])  [unwired: 3 in, 1 out]
      n177 = Index Array(array=w527, index=0) -> (element=w525:dbl)
    }
    frame "StringMD5" {
      n178 = Unbundle By Name(w556) -> ("StringMD5"=w555:T4)
      n179 = call <vilib>:"Unflatten From JSON String.vi"("Type and Defaults"=w555, "error in (no error)"=w560, "JSON String"=w561) -> ("error out"=w563:errorcluster, "Variant"=w564:variant)  [unwired: 7 in]
      n180 = Variant To Data(error in=w563, type=w555, Variant=w564) -> (data=w562:T4, error out=w550:errorcluster)
      n181 = Unbundle By Name(w562) -> ("json.StringVar"=w551:string)
      n182 = Empty String/Path?(string/path=w551) -> (empty?=w553:bool)
      n183 = case shown="False" w553 {
        tunnel: w550 -> [w573 w578]
        tunnel: w552 -> [w569 _]
        tunnel: [w565 w574] -> w547
        tunnel: w551 -> [w571 _]
        tunnel: [w567 w576] -> w548
        tunnel: w549 -> [w568 w575]
        frame False {
          n184 = call "StringVariableParse.vi"("error in"=w573, "Info"=w568, "in"=w571, "dictionary"=w569) -> ("error out"=w565:errorcluster, "out"=w566:string)  [unwired: 5 in, 1 out]
          n185 = Concatenate Strings("String：" ("string"), w566) -> (w572:string)
          n186 = call "Log.vi"("error in"=w565, "LogIn"=w572, "Info"=w568) -> ()  [unwired: 9 in]
          n187 = call-poly <userlib>:"MD5 Message Digest__ogtk.vi"("Message"=w566) -> ("MD5 Message Digest"=w567:string)
        }
        frame True {
          w576 = "变量名为空" ("source")
          n188 = Bundle By Name(cluster=w578, "source"=w576, "status"=TRUE) -> (w574:errorcluster)
          n189 = call "Log.vi"("error in"=w574, "Info"=w575) -> ()  [unwired: 10 in]
        }
      }
      n190 = Build Array(w548) -> (w554:string[])
      n191 = Fract/Exp String To Number(string=w554) -> (number=w559:dbl[])  [unwired: 3 in, 1 out]
      n192 = Index Array(array=w559, index=0) -> (element=w557:dbl)
    }
    frame "NumStringToHexString" {
      n193 = Unbundle By Name(w588) -> ("NumStringToHexString"=w587:T4)
      n194 = call <vilib>:"Unflatten From JSON String.vi"("Type and Defaults"=w587, "error in (no error)"=w592, "JSON String"=w593) -> ("error out"=w595:errorcluster, "Variant"=w596:variant)  [unwired: 7 in]
      n195 = Variant To Data(error in=w595, type=w587, Variant=w596) -> (data=w594:T4, error out=w582:errorcluster)
      n196 = Unbundle By Name(w594) -> ("json.StringVar"=w583:string)
      n197 = Empty String/Path?(string/path=w583) -> (empty?=w585:bool)
      n198 = case shown="False" w585 {
        tunnel: w582 -> [w606 w611]
        tunnel: w584 -> [w602 _]
        tunnel: [w600 w607] -> w579
        tunnel: w583 -> [w604 _]
        tunnel: [w597 w609] -> w580
        tunnel: w581 -> [w601 w608]
        frame False {
          n199 = call "StringVariableParse.vi"("error in"=w606, "Info"=w601, "in"=w604, "dictionary"=w602) -> ("error out"=w600:errorcluster, "out"=w598:string)  [unwired: 5 in, 1 out]
          n200 = Decimal String To Number(string=w598) -> (number=w599:i32)  [unwired: 2 in, 1 out]
          n201 = Concatenate Strings("String：" ("string"), w598) -> (w605:string)
          n202 = call "Log.vi"("error in"=w600, "LogIn"=w605, "Info"=w601) -> ()  [unwired: 9 in]
          n203 = Number To Hexadecimal String(2:w599) -> (0:w597:string)  [unwired: 1 in]
        }
        frame True {
          w609 = "变量名为空" ("source")
          n204 = Bundle By Name(cluster=w611, "source"=w609, "status"=TRUE) -> (w607:errorcluster)
          n205 = call "Log.vi"("error in"=w607, "Info"=w608) -> ()  [unwired: 10 in]
        }
      }
      n206 = Build Array(w580) -> (w586:string[])
      n207 = Fract/Exp String To Number(string=w586) -> (number=w591:dbl[])  [unwired: 3 in, 1 out]
      n208 = Index Array(array=w591, index=0) -> (element=w589:dbl)
    }
    frame "HexStringToNumString" {
      n209 = Unbundle By Name(w621) -> ("HexStringToNumString"=w620:T4)
      n210 = call <vilib>:"Unflatten From JSON String.vi"("Type and Defaults"=w620, "error in (no error)"=w625, "JSON String"=w626) -> ("error out"=w628:errorcluster, "Variant"=w629:variant)  [unwired: 7 in]
      n211 = Variant To Data(error in=w628, type=w620, Variant=w629) -> (data=w627:T4, error out=w615:errorcluster)
      n212 = Unbundle By Name(w627) -> ("json.StringVar"=w616:string)
      n213 = Empty String/Path?(string/path=w616) -> (empty?=w618:bool)
      n214 = case shown="False" w618 {
        tunnel: w615 -> [w639 w644]
        tunnel: w617 -> [w635 _]
        tunnel: [w633 w640] -> w612
        tunnel: w616 -> [w637 _]
        tunnel: [w630 w642] -> w613
        tunnel: w614 -> [w634 w641]
        frame False {
          n215 = call "StringVariableParse.vi"("error in"=w639, "Info"=w634, "in"=w637, "dictionary"=w635) -> ("error out"=w633:errorcluster, "out"=w631:string)  [unwired: 5 in, 1 out]
          n216 = Hexadecimal String To Number(string=w631) -> (number=w632:u32)  [unwired: 2 in, 1 out]
          n217 = Concatenate Strings("String：" ("string"), w631) -> (w638:string)
          n218 = call "Log.vi"("error in"=w633, "LogIn"=w638, "Info"=w634) -> ()  [unwired: 9 in]
          n219 = Number To Decimal String(number=w632) -> (decimal integer string=w630:string)  [unwired: 1 in]
        }
        frame True {
          w642 = "变量名为空" ("source")
          n220 = Bundle By Name(cluster=w644, "source"=w642, "status"=TRUE) -> (w640:errorcluster)
          n221 = call "Log.vi"("error in"=w640, "Info"=w641) -> ()  [unwired: 10 in]
        }
      }
      n222 = Build Array(w613) -> (w619:string[])
      n223 = Fract/Exp String To Number(string=w619) -> (number=w624:dbl[])  [unwired: 3 in, 1 out]
      n224 = Index Array(array=w624, index=0) -> (element=w622:dbl)
    }
    frame "StartWith" {
      n225 = Unbundle By Name(w656) -> ("StartWith"=w655:T14)
      n226 = call <vilib>:"Unflatten From JSON String.vi"("Type and Defaults"=w655, "error in (no error)"=w660, "JSON String"=w661) -> ("error out"=w663:errorcluster, "Variant"=w664:variant)  [unwired: 7 in]
      n227 = Variant To Data(error in=w663, type=w655, Variant=w664) -> (data=w662:T14, error out=w650:errorcluster)
      n228 = Unbundle By Name(w662) -> ("json.StringVar"=w651:string, "json.SubString"=w646:string, "json.IgnoreCasse"=w645:bool)
      n229 = Empty String/Path?(string/path=w651) -> (empty?=w653:bool)
      n230 = case shown="False" w653 {
        tunnel: w650 -> [w683 w804]
        tunnel: w652 -> [w673 _]
        tunnel: [w668 w800] -> w647
        tunnel: w651 -> [w681 _]
        tunnel: [w667 w802] -> w648
        tunnel: w649 -> [w671 w801]
        tunnel: w646 -> [w672 _]
        tunnel: w645 -> [w670 _]
        frame False {
          n231 = call "StringVariableParse.vi"("error in"=w683, "Info"=w671, "in"=w681, "dictionary"=w673) -> ("error out"=w674:errorcluster, "out"=w675:string)  [unwired: 5 in, 1 out]
          n232 = call "StringVariableParse.vi"("error in"=w674, "Info"=w671, "in"=w672, "dictionary"=w673) -> ("error out"=w669:errorcluster, "out"=w665:string)  [unwired: 5 in, 1 out]
          n233 = Concatenate Strings("^" ("string"), w665) -> (w679:string)
          n234 = Concatenate Strings("String：" ("string"), w675, "Substring：" ("string"), w665) -> (w682:string)
          n235 = call "Log.vi"("error in"=w669, "LogIn"=w682, "Info"=w671) -> ()  [unwired: 9 in]
          n236 = xnode "Match Regular Expression"("input string"=w675, "regular expression"=w679, "ignore case? (F)"=w670) -> ("whole match"=w667:string, "offset past match"=w677:i32)  [unwired: 3 in, 3 out]
          n237 = Greater Or Equal To 0?(x=w677) -> (x >= 0?=w676:bool)
          n238 = in-place {
            in-place-border: w676 -> [w799]
            n239 = in-place-cluster #1(w669) -> ()  [unwired: 1 out]
            n240 = Not(x=w799) -> (.not. x?=w798:bool)
            n241 = in-place-cluster #1("status"=w798) -> (w668:errorcluster)
          }
        }
        frame True {
          w802 = "变量名为空" ("source")
          n242 = Bundle By Name(cluster=w804, "source"=w802, "status"=TRUE) -> (w800:errorcluster)
          n243 = call "Log.vi"("error in"=w800, "Info"=w801) -> ()  [unwired: 10 in]
        }
      }
      n244 = Build Array(w648) -> (w654:string[])
      n245 = Fract/Exp String To Number(string=w654) -> (number=w659:dbl[])  [unwired: 3 in, 1 out]
      n246 = Index Array(array=w659, index=0) -> (element=w657:dbl)
    }
    frame "EndWith" {
      n247 = Unbundle By Name(w816) -> ("EndWith"=w815:T14)
      n248 = call <vilib>:"Unflatten From JSON String.vi"("Type and Defaults"=w815, "error in (no error)"=w820, "JSON String"=w821) -> ("error out"=w823:errorcluster, "Variant"=w824:variant)  [unwired: 7 in]
      n249 = Variant To Data(error in=w823, type=w815, Variant=w824) -> (data=w822:T14, error out=w810:errorcluster)
      n250 = Unbundle By Name(w822) -> ("json.StringVar"=w811:string, "json.SubString"=w806:string, "json.IgnoreCasse"=w805:bool)
      n251 = Empty String/Path?(string/path=w811) -> (empty?=w813:bool)
      n252 = case shown="False" w813 {
        tunnel: w810 -> [w843 w964]
        tunnel: w812 -> [w835 _]
        tunnel: [w830 w960] -> w807
        tunnel: w811 -> [w841 _]
        tunnel: [w829 w962] -> w808
        tunnel: w809 -> [w833 w961]
        tunnel: w806 -> [w834 _]
        tunnel: w805 -> [w832 _]
        frame False {
          n253 = call "StringVariableParse.vi"("error in"=w843, "Info"=w833, "in"=w841, "dictionary"=w835) -> ("error out"=w836:errorcluster, "out"=w837:string)  [unwired: 5 in, 1 out]
          n254 = call "StringVariableParse.vi"("error in"=w836, "Info"=w833, "in"=w834, "dictionary"=w835) -> ("error out"=w831:errorcluster, "out"=w825:string)  [unwired: 5 in, 1 out]
          n255 = Concatenate Strings(w825, "$" ("string")) -> (w827:string)
          n256 = Concatenate Strings("String：" ("string"), w837, "Substring：" ("string"), w825) -> (w842:string)
          n257 = call "Log.vi"("error in"=w831, "LogIn"=w842, "Info"=w833) -> ()  [unwired: 9 in]
          n258 = xnode "Match Regular Expression"("input string"=w837, "regular expression"=w827, "ignore case? (F)"=w832) -> ("whole match"=w829:string, "offset past match"=w839:i32)  [unwired: 3 in, 3 out]
          n259 = Greater Or Equal To 0?(x=w839) -> (x >= 0?=w838:bool)
          n260 = in-place {
            in-place-border: w838 -> [w959]
            n261 = in-place-cluster #2(w831) -> ()  [unwired: 1 out]
            n262 = Not(x=w959) -> (.not. x?=w958:bool)
            n263 = in-place-cluster #2("status"=w958) -> (w830:errorcluster)
          }
        }
        frame True {
          w962 = "变量名为空" ("source")
          n264 = Bundle By Name(cluster=w964, "source"=w962, "status"=TRUE) -> (w960:errorcluster)
          n265 = call "Log.vi"("error in"=w960, "Info"=w961) -> ()  [unwired: 10 in]
        }
      }
      n266 = Build Array(w808) -> (w814:string[])
      n267 = Fract/Exp String To Number(string=w814) -> (number=w819:dbl[])  [unwired: 3 in, 1 out]
      n268 = Index Array(array=w819, index=0) -> (element=w817:dbl)
    }
    frame "AfterSubstring" {
      n269 = Unbundle By Name(w975) -> ("AfterSubstring"=w974:T15)
      n270 = call <vilib>:"Unflatten From JSON String.vi"("Type and Defaults"=w974, "error in (no error)"=w979, "JSON String"=w980) -> ("error out"=w982:errorcluster, "Variant"=w983:variant)  [unwired: 7 in]
      n271 = Variant To Data(error in=w982, type=w974, Variant=w983) -> (data=w981:T15, error out=w969:errorcluster)
      n272 = Unbundle By Name(w981) -> ("json.StringVar"=w970:string, "json.SubString"=w965:string)
      n273 = Empty String/Path?(string/path=w970) -> (empty?=w972:bool)
      n274 = case shown="False" w972 {
        tunnel: w969 -> [w995 w1000]
        tunnel: w971 -> [w989 _]
        tunnel: [w984 w996] -> w966
        tunnel: w970 -> [w993 _]
        tunnel: [w985 w998] -> w967
        tunnel: w968 -> [w987 w997]
        tunnel: w965 -> [w988 _]
        frame False {
          n275 = call "StringVariableParse.vi"("error in"=w995, "Info"=w987, "in"=w993, "dictionary"=w989) -> ("error out"=w990:errorcluster, "out"=w991:string)  [unwired: 5 in, 1 out]
          n276 = Concatenate Strings("String：" ("string"), w991) -> (w994:string)
          n277 = call "StringVariableParse.vi"("error in"=w990, "Info"=w987, "in"=w988, "dictionary"=w989) -> ("error out"=w984:errorcluster, "out"=w986:string)  [unwired: 5 in, 1 out]
          n278 = call "Log.vi"("error in"=w984, "LogIn"=w994, "Info"=w987) -> ()  [unwired: 9 in]
          n279 = Match Pattern(string=w991, regular expression=w986) -> (after substring=w985:string)  [unwired: 1 in, 3 out]
        }
        frame True {
          w998 = "变量名为空" ("source")
          n280 = Bundle By Name(cluster=w1000, "source"=w998, "status"=TRUE) -> (w996:errorcluster)
          n281 = call "Log.vi"("error in"=w996, "Info"=w997) -> ()  [unwired: 10 in]
        }
      }
      n282 = Build Array(w967) -> (w973:string[])
      n283 = Fract/Exp String To Number(string=w973) -> (number=w978:dbl[])  [unwired: 3 in, 1 out]
      n284 = Index Array(array=w978, index=0) -> (element=w976:dbl)
    }
    frame "BeforeSubstring" {
      n285 = Unbundle By Name(w1011) -> ("BeforeSubstring"=w1010:T15)
      n286 = call <vilib>:"Unflatten From JSON String.vi"("Type and Defaults"=w1010, "error in (no error)"=w1015, "JSON String"=w1016) -> ("error out"=w1018:errorcluster, "Variant"=w1019:variant)  [unwired: 7 in]
      n287 = Variant To Data(error in=w1018, type=w1010, Variant=w1019) -> (data=w1017:T15, error out=w1006:errorcluster)
      n288 = Unbundle By Name(w1017) -> ("json.StringVar"=w1007:string, "json.SubString"=w1003:string)
      n289 = Empty String/Path?(string/path=w1007) -> (empty?=w1009:bool)
      n290 = case shown="False" w1009 {
        tunnel: w1006 -> [w1031 w1036]
        tunnel: w1008 -> [w1025 _]
        tunnel: [w1021 w1032] -> w1004
        tunnel: w1007 -> [w1029 _]
        tunnel: [w1020 w1034] -> w1002
        tunnel: w1005 -> [w1023 w1033]
        tunnel: w1003 -> [w1024 _]
        frame False {
          n291 = call "StringVariableParse.vi"("error in"=w1031, "Info"=w1023, "in"=w1029, "dictionary"=w1025) -> ("error out"=w1026:errorcluster, "out"=w1027:string)  [unwired: 5 in, 1 out]
          n292 = Concatenate Strings("String：" ("string"), w1027) -> (w1030:string)
          n293 = call "StringVariableParse.vi"("error in"=w1026, "Info"=w1023, "in"=w1024, "dictionary"=w1025) -> ("error out"=w1021:errorcluster, "out"=w1022:string)  [unwired: 5 in, 1 out]
          n294 = call "Log.vi"("error in"=w1021, "LogIn"=w1030, "Info"=w1023) -> ()  [unwired: 9 in]
          n295 = Match Pattern(string=w1027, regular expression=w1022) -> (before substring=w1020:string)  [unwired: 1 in, 3 out]
        }
        frame True {
          w1034 = "变量名为空" ("source")
          n296 = Bundle By Name(cluster=w1036, "source"=w1034, "status"=TRUE) -> (w1032:errorcluster)
          n297 = call "Log.vi"("error in"=w1032, "Info"=w1033) -> ()  [unwired: 10 in]
        }
      }
      n298 = Build Array(w1002) -> (w1001:string[])
      n299 = Fract/Exp String To Number(string=w1001) -> (number=w1014:dbl[])  [unwired: 3 in, 1 out]
      n300 = Index Array(array=w1014, index=0) -> (element=w1012:dbl)
    }
    frame "MiddleSubstring" {
      n301 = Unbundle By Name(w1048) -> ("MiddleSubstring"=w1047:T16)
      n302 = call <vilib>:"Unflatten From JSON String.vi"("Type and Defaults"=w1047, "error in (no error)"=w1052, "JSON String"=w1053) -> ("error out"=w1055:errorcluster, "Variant"=w1056:variant)  [unwired: 7 in]
      n303 = Variant To Data(error in=w1055, type=w1047, Variant=w1056) -> (data=w1054:T16, error out=w1043:errorcluster)
      n304 = Unbundle By Name(w1054) -> ("json.StringVar"=w1044:string, "json.BeforeSubString"=w1040:string, "json.AfterSubString"=w1039:string)
      n305 = Empty String/Path?(string/path=w1044) -> (empty?=w1046:bool)
      n306 = case shown="True" w1046 {
        tunnel: w1043 -> [w1071 w1088]
        tunnel: w1045 -> [w1062 _]
        tunnel: [w1059 w1084] -> w1041
        tunnel: w1044 -> [w1069 _]
        tunnel: [w1057 w1083] -> w1038
        tunnel: w1042 -> [w1060 w1085]
        tunnel: w1040 -> [w1065 _]
        tunnel: w1039 -> [w1061 _]
        frame False {
          n307 = call "StringVariableParse.vi"("error in"=w1071, "Info"=w1060, "in"=w1069, "dictionary"=w1062) -> ("error out"=w1066:errorcluster, "out"=w1067:string)  [unwired: 5 in, 1 out]
          n308 = call "StringVariableParse.vi"("error in"=w1066, "Info"=w1060, "in"=w1065, "dictionary"=w1062) -> ("error out"=w1063:errorcluster, "out"=w1064:string)  [unwired: 5 in, 1 out]
          n309 = Concatenate Strings("String：" ("string"), w1067) -> (w1070:string)
          n310 = call "StringVariableParse.vi"("error in"=w1063, "Info"=w1060, "in"=w1061, "dictionary"=w1062) -> ("error out"=w1059:errorcluster, "out"=w1058:string)  [unwired: 5 in, 1 out]
          n311 = while {
            tunnel: w1058 -> [w1079]
            tunnel: w1064 -> [w1081]
            tunnel: [w1078] -> w1057 mode=indexing if=w1073
            shift-right: [w1072] -> _
            shift-left: w1067 -> [w1082]
            stop <- w1073 continue-if-true
            n312 = Match Pattern(string=w1082, regular expression=w1081) -> (after substring=w1080:string, offset past match=w1077:i32)  [unwired: 1 in, 2 out]
            n313 = Match Pattern(string=w1080, regular expression=w1079) -> (before substring=w1078:string, after substring=w1072:string, offset past match=w1076:i32)  [unwired: 1 in, 1 out]
            n314 = Greater Or Equal To 0?(x=w1076) -> (x >= 0?=w1075:bool)
            n315 = Greater Or Equal To 0?(x=w1077) -> (x >= 0?=w1074:bool)
            n316 = And(x=w1075, y=w1074) -> (x .and. y?=w1073:bool)
          }
          n317 = call "Log.vi"("error in"=w1059, "LogIn"=w1070, "Info"=w1060) -> ()  [unwired: 9 in]
        }
        frame True {
          w1086 = "变量名为空" ("source")
          n318 = Bundle By Name(cluster=w1088, "source"=w1086, "status"=TRUE) -> (w1084:errorcluster)
          n319 = call "Log.vi"("error in"=w1084, "Info"=w1085) -> ()  [unwired: 10 in]
          n320 = Build Array(w1086) -> (w1083:string[])
        }
      }
      n321 = Index Array(array=w1038) -> (element=w1037:string)  [unwired: 1 in]
      n322 = Fract/Exp String To Number(string=w1038) -> (number=w1051:dbl[])  [unwired: 3 in, 1 out]
      n323 = Index Array(array=w1051, index=0) -> (element=w1049:dbl)
    }
    frame "AsciiToHexString" {
      n324 = Unbundle By Name(w1098) -> ("AsciiToHexString"=w1097:T4)
      n325 = call <vilib>:"Unflatten From JSON String.vi"("Type and Defaults"=w1097, "error in (no error)"=w1102, "JSON String"=w1103) -> ("error out"=w1105:errorcluster, "Variant"=w1106:variant)  [unwired: 7 in]
      n326 = Variant To Data(error in=w1105, type=w1097, Variant=w1106) -> (data=w1104:T4, error out=w1093:errorcluster)
      n327 = Unbundle By Name(w1104) -> ("json.StringVar"=w1094:string)
      n328 = Empty String/Path?(string/path=w1094) -> (empty?=w1096:bool)
      n329 = case shown="False" w1096 {
        tunnel: w1093 -> [w1119 w1135]
        tunnel: w1095 -> [w1115 _]
        tunnel: [w1107 w1131] -> w1091
        tunnel: w1094 -> [w1117 _]
        tunnel: [w1108 w1133] -> w1089
        tunnel: w1092 -> [w1114 w1132]
        frame False {
          n330 = call "StringVariableParse.vi"("error in"=w1119, "Info"=w1114, "in"=w1117, "dictionary"=w1115) -> ("error out"=w1107:errorcluster, "out"=w1109:string)  [unwired: 5 in, 1 out]
          n331 = String Length(string=w1109) -> (length=w1111:i32)
          n332 = Concatenate Strings("String：" ("string"), w1109) -> (w1118:string)
          n333 = Quotient & Remainder(x=w1111, y=2) -> (floor(x/y)=w1112:i32)  [unwired: 1 out]
          n334 = call "Log.vi"("error in"=w1107, "LogIn"=w1118, "Info"=w1114) -> ()  [unwired: 9 in]
          n335 = for {
            N: w1112 -> [_]
            tunnel: w1109 -> [w1130]
            shift-right: [w1122] -> w1108
            shift-left: "" -> [w1121]
            i -> [w1127]
            w1128 = 2 ("length (rest)")
            n336 = Multiply(x=w1127, y=w1128) -> (x*y=w1129:i32)
            n337 = String Subset(string=w1130, offset (0)=w1129, length (rest)=w1128) -> (substring=w1126:string)
            n338 = Hexadecimal String To Number(string=w1126) -> (number=w1125:u32)  [unwired: 2 in, 1 out]
            n339 = To Unsigned Byte Integer(number=w1125) -> (unsigned 8bit integer=w1124:u8)
            n340 = Type Cast(type="", x=w1124) -> (*(type *) &x=w1120:string)
            n341 = Concatenate Strings(w1121, w1120) -> (w1122:string)
          }
        }
        frame True {
          w1133 = "变量名为空" ("source")
          n342 = Bundle By Name(cluster=w1135, "source"=w1133, "status"=TRUE) -> (w1131:errorcluster)
          n343 = call "Log.vi"("error in"=w1131, "Info"=w1132) -> ()  [unwired: 10 in]
        }
      }
      n344 = Build Array(w1089) -> (w1090:string[])
      n345 = Fract/Exp String To Number(string=w1090) -> (number=w1101:dbl[])  [unwired: 3 in, 1 out]
      n346 = Index Array(array=w1101, index=0) -> (element=w1099:dbl)
    }
    frame "HexStringToAscii" {
      n347 = Unbundle By Name(w1145) -> ("HexStringToAscii"=w1144:T4)
      n348 = call <vilib>:"Unflatten From JSON String.vi"("Type and Defaults"=w1144, "error in (no error)"=w1149, "JSON String"=w1150) -> ("error out"=w1152:errorcluster, "Variant"=w1153:variant)  [unwired: 7 in]
      n349 = Variant To Data(error in=w1152, type=w1144, Variant=w1153) -> (data=w1151:T4, error out=w1140:errorcluster)
      n350 = Unbundle By Name(w1151) -> ("json.StringVar"=w1141:string)
      n351 = Empty String/Path?(string/path=w1141) -> (empty?=w1143:bool)
      n352 = case shown="False" w1143 {
        tunnel: w1140 -> [w1164 w1178]
        tunnel: w1142 -> [w1160 _]
        tunnel: [w1158 w1174] -> w1138
        tunnel: w1141 -> [w1162 _]
        tunnel: [w1154 w1176] -> w1136
        tunnel: w1139 -> [w1159 w1175]
        frame False {
          n353 = call "StringVariableParse.vi"("error in"=w1164, "Info"=w1159, "in"=w1162, "dictionary"=w1160) -> ("error out"=w1158:errorcluster, "out"=w1155:string)  [unwired: 5 in, 1 out]
          n354 = String Length(string=w1155) -> (length=w1157:i32)
          n355 = Concatenate Strings("String：" ("string"), w1155) -> (w1163:string)
          n356 = for {
            N: w1157 -> [_]
            tunnel: w1155 -> [w1173]
            shift-right: [w1168] -> w1154
            shift-left: "" -> [w1167]
            i -> [w1172]
            w1170 = u8 1 ("length (rest)")
            n357 = String Subset(string=w1173, offset (0)=w1172, length (rest)=w1170) -> (substring=w1171:string)
            n358 = Type Cast(type=w1170, x=w1171) -> (*(type *) &x=w1169:u8)
            n359 = Number To Hexadecimal String(1:i16 2 ("width (-)"), 2:w1169) -> (0:w1166:string)
            n360 = Concatenate Strings(w1167, w1166) -> (w1168:string)
          }
          n361 = call "Log.vi"("error in"=w1158, "LogIn"=w1163, "Info"=w1159) -> ()  [unwired: 9 in]
        }
        frame True {
          w1176 = "变量名为空" ("source")
          n362 = Bundle By Name(cluster=w1178, "source"=w1176, "status"=TRUE) -> (w1174:errorcluster)
          n363 = call "Log.vi"("error in"=w1174, "Info"=w1175) -> ()  [unwired: 10 in]
        }
      }
      n364 = Build Array(w1136) -> (w1137:string[])
      n365 = Fract/Exp String To Number(string=w1137) -> (number=w1148:dbl[])  [unwired: 3 in, 1 out]
      n366 = Index Array(array=w1148, index=0) -> (element=w1146:dbl)
    }
    frame "StringTo1DArray" {
      n367 = Unbundle By Name(w1189) -> ("StringTo1DArray"=w1188:T17)
      n368 = call <vilib>:"Unflatten From JSON String.vi"("Type and Defaults"=w1188, "error in (no error)"=w1193, "JSON String"=w1194) -> ("error out"=w1196:errorcluster, "Variant"=w1197:variant)  [unwired: 7 in]
      n369 = Variant To Data(error in=w1196, type=w1188, Variant=w1197) -> (data=w1195:T17, error out=w1184:errorcluster)
      n370 = Unbundle By Name(w1195) -> ("json.StringVar"=w1185:string, "json.Delimiter"=w1181:string)
      n371 = Empty String/Path?(string/path=w1185) -> (empty?=w1187:bool)
      n372 = case shown="True" w1187 {
        tunnel: w1184 -> [w1210 w1216]
        tunnel: w1186 -> [w1205 _]
        tunnel: [w1201 w1212] -> w1182
        tunnel: w1185 -> [w1208 _]
        tunnel: [w1200 w1211] -> w1179
        tunnel: w1183 -> [w1202 w1213]
        tunnel: w1181 -> [w1204 _]
        frame False {
          n373 = call "StringVariableParse.vi"("error in"=w1210, "Info"=w1202, "in"=w1208, "dictionary"=w1205) -> ("error out"=w1203:errorcluster, "out"=w1206:string)  [unwired: 5 in, 1 out]
          n374 = call "StringVariableParse.vi"("error in"=w1203, "Info"=w1202, "in"=w1204, "dictionary"=w1205) -> ("error out"=w1201:errorcluster, "out"=w1198:string)  [unwired: 5 in, 1 out]
          n375 = call <userlib>:"String to 1D Array__ogtk.vi"("delimiter (Tab)"=w1198, "string"=w1206) -> ("Array of Strings"=w1200:string[])  [unwired: 9 in]
          n376 = Concatenate Strings("String：" ("string"), w1206, "Delimiter：" ("string"), w1198) -> (w1209:string)
          n377 = call "Log.vi"("error in"=w1201, "LogIn"=w1209, "Info"=w1202) -> ()  [unwired: 9 in]
        }
        frame True {
          w1214 = "变量名为空" ("source")
          n378 = Bundle By Name(cluster=w1216, "source"=w1214, "status"=TRUE) -> (w1212:errorcluster)
          n379 = call "Log.vi"("error in"=w1212, "Info"=w1213) -> ()  [unwired: 10 in]
          n380 = Build Array(w1214) -> (w1211:string[])
        }
      }
      n381 = Index Array(array=w1179) -> (element=w1180:string)  [unwired: 1 in]
      n382 = Fract/Exp String To Number(string=w1179) -> (number=w1192:dbl[])  [unwired: 3 in, 1 out]
      n383 = Index Array(array=w1192, index=0) -> (element=w1190:dbl)
    }
    frame "StringToCharacterArray" {
      n384 = Unbundle By Name(w1226) -> ("StringToCharacterArray"=w1225:T4)
      n385 = call <vilib>:"Unflatten From JSON String.vi"("Type and Defaults"=w1225, "error in (no error)"=w1230, "JSON String"=w1231) -> ("error out"=w1233:errorcluster, "Variant"=w1234:variant)  [unwired: 7 in]
      n386 = Variant To Data(error in=w1233, type=w1225, Variant=w1234) -> (data=w1232:T4, error out=w1221:errorcluster)
      n387 = Unbundle By Name(w1232) -> ("json.StringVar"=w1222:string)
      n388 = Empty String/Path?(string/path=w1222) -> (empty?=w1224:bool)
      n389 = case shown="False" w1224 {
        tunnel: w1221 -> [w1243 w1249]
        tunnel: w1223 -> [w1239 _]
        tunnel: [w1237 w1245] -> w1219
        tunnel: w1222 -> [w1241 _]
        tunnel: [w1235 w1244] -> w1217
        tunnel: w1220 -> [w1238 w1246]
        frame False {
          n390 = call "StringVariableParse.vi"("error in"=w1243, "Info"=w1238, "in"=w1241, "dictionary"=w1239) -> ("error out"=w1237:errorcluster, "out"=w1236:string)  [unwired: 5 in, 1 out]
          n391 = Concatenate Strings("String：" ("string"), w1236) -> (w1242:string)
          n392 = call "Log.vi"("error in"=w1237, "LogIn"=w1242, "Info"=w1238) -> ()  [unwired: 9 in]
          n393 = call <userlib>:"String to Character Array__ogtk.vi"("Input String"=w1236) -> ("Character Array"=w1235:string[])
        }
        frame True {
          w1247 = "变量名为空" ("source")
          n394 = Bundle By Name(cluster=w1249, "source"=w1247, "status"=TRUE) -> (w1245:errorcluster)
          n395 = call "Log.vi"("error in"=w1245, "Info"=w1246) -> ()  [unwired: 10 in]
          n396 = Build Array(w1247) -> (w1244:string[])
        }
      }
      n397 = Index Array(array=w1217) -> (element=w1218:string)  [unwired: 1 in]
      n398 = Fract/Exp String To Number(string=w1217) -> (number=w1229:dbl[])  [unwired: 3 in, 1 out]
      n399 = Index Array(array=w1229, index=0) -> (element=w1227:dbl)
    }
    frame "RemoveAllWhitespace" {
      n400 = Unbundle By Name(w1259) -> ("RemoveAllWhitespace"=w1258:T4)
      n401 = call <vilib>:"Unflatten From JSON String.vi"("Type and Defaults"=w1258, "error in (no error)"=w1263, "JSON String"=w1264) -> ("error out"=w1266:errorcluster, "Variant"=w1267:variant)  [unwired: 7 in]
      n402 = Variant To Data(error in=w1266, type=w1258, Variant=w1267) -> (data=w1265:T4, error out=w1254:errorcluster)
      n403 = Unbundle By Name(w1265) -> ("json.StringVar"=w1255:string)
      n404 = Empty String/Path?(string/path=w1255) -> (empty?=w1257:bool)
      n405 = case shown="False" w1257 {
        tunnel: w1254 -> [w1276 w1281]
        tunnel: w1256 -> [w1272 _]
        tunnel: [w1270 w1278] -> w1252
        tunnel: w1255 -> [w1274 _]
        tunnel: [w1268 w1277] -> w1250
        tunnel: w1253 -> [w1271 w1279]
        frame False {
          n406 = call "StringVariableParse.vi"("error in"=w1276, "Info"=w1271, "in"=w1274, "dictionary"=w1272) -> ("error out"=w1270:errorcluster, "out"=w1269:string)  [unwired: 5 in, 1 out]
          n407 = Concatenate Strings("String：" ("string"), w1269) -> (w1275:string)
          n408 = call "Log.vi"("error in"=w1270, "LogIn"=w1275, "Info"=w1271) -> ()  [unwired: 9 in]
          n409 = call <userlib>:"MGI Remove All Whitespace.vi"("String"=w1269) -> ("Trimmed String"=w1268:string)
        }
        frame True {
          w1277 = "变量名为空" ("source")
          n410 = Bundle By Name(cluster=w1281, "source"=w1277, "status"=TRUE) -> (w1278:errorcluster)
          n411 = call "Log.vi"("error in"=w1278, "Info"=w1279) -> ()  [unwired: 10 in]
        }
      }
      n412 = Build Array(w1250) -> (w1251:string[])
      n413 = Fract/Exp String To Number(string=w1251) -> (number=w1262:dbl[])  [unwired: 3 in, 1 out]
      n414 = Index Array(array=w1262, index=0) -> (element=w1260:dbl)
    }
  }
  "StrResult" <- w12
  "Error Out" <- w14
  "StrResultArray" <- w11
  "NumResult" <- w10
  "NumResultArray" <- w9
